vi "Read Enabled Values.vi"(8 "error in (no error)":errorcluster, 11 "Single Channel  in":refnum<class "Single Channel.lvclass">) -> (0 "error out":errorcluster, 2 "Data Values":dbl[](array[numeric]), 3 "Single Channel out":refnum<class "Single Channel.lvclass">)   [LabVIEW 2018, in "Single Channel.lvclass"]
uses:
  Single Channel.lvclass
  Single Channel.lvclass/Single Channel.ctl
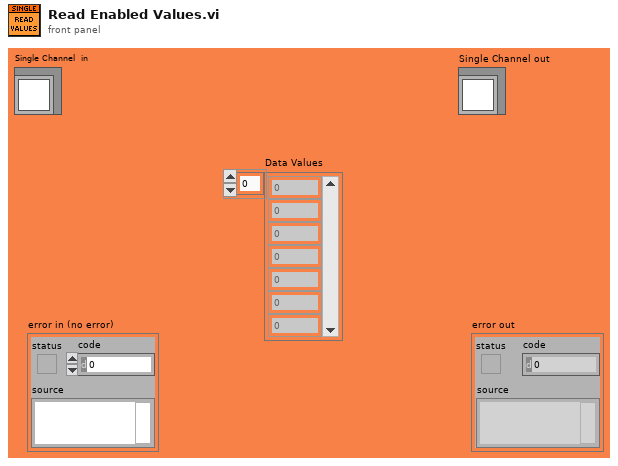
[diagram p1: front panel]
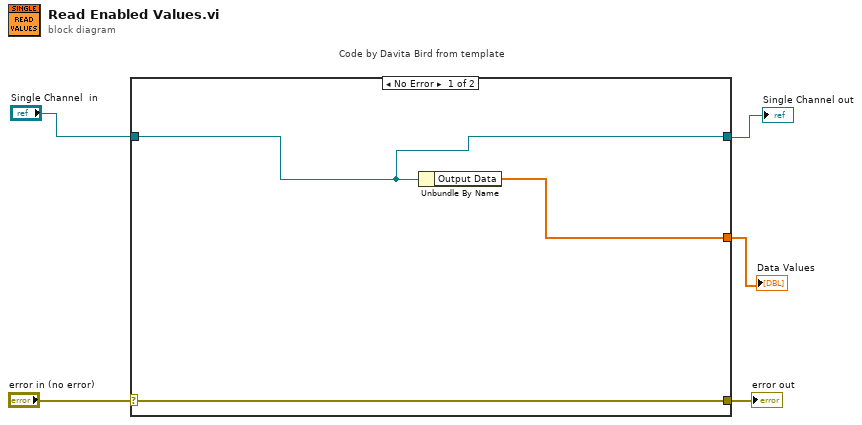
[diagram p0: block diagram]
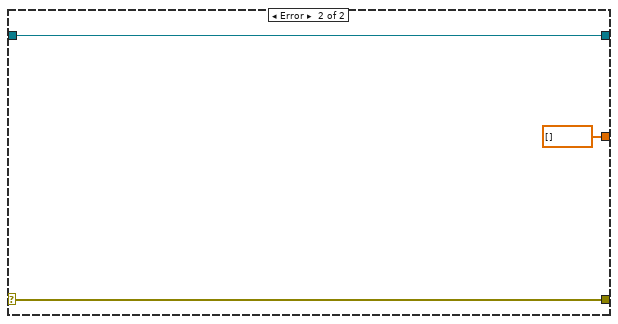
[diagram p2: hidden frame]
diagram:
  n1 = case "Code by Davita Bird from template" shown="No Error" "error in (no error)" {
    selector: "error in (no error)" -> [w8 w11]
    tunnel: [w8 w11] -> w4
    tunnel: [w7 w10] -> w1
    tunnel: "Single Channel  in" -> [w7 w10]
    tunnel: [w6 dbl[] [] ("array type (2D Dbl)")] -> w3
    frame No Error {
      n2 = Unbundle By Name(w7) -> ("Output Data"=w6:dbl[])
    }
    frame Error {
    }
  }
  "error out" <- w4
  "Data Values" <- w3
  "Single Channel out" <- w1
